vi "read.vi"(8 "error in (no error)":errorcluster, 10 "ILC":refnum<class "ILC.lvclass">, 11 "ReadILCTachometerStrategy in":refnum<class "ReadILCTachometerStrategy.lvclass">) -> (0 "error out":errorcluster, 2 "Value":dbl, 3 "ReadILCTachometerStrategy out":refnum<class "ReadILCTachometerStrategy.lvclass">)   [LabVIEW 2016, in "ReadILCTachometerStrategy.lvclass"]
uses:
  ReadILCTachometerStrategy.lvclass
  Common_ILC/ILC/ILC.lvclass
  Common_ILC/ILC/ILC.lvclass/ILC.ctl
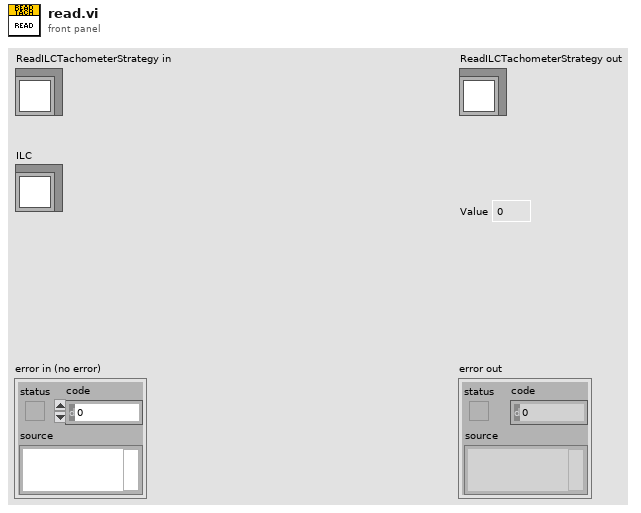
[diagram p1: front panel]
types:
  T1 = typedef "ILCCommon.lvlib/ILCTypedefs.lvlib/Inputs.ctl" = cluster{"Input Channels":T2, "Limit Switches":T3, "Tachometer":u16, "SSI Encoder":i32, "ADC":T4}
  T2 = typedef "ILCCommon.lvlib/ILCConfiguration.lvlib/Input Channels.ctl" = enum16{"Channel 0", "3 Channels", "5 Channels"}
  T3 = typedef "ILCCommon.lvlib/ILCTypedefs.lvlib/Limit Switches.ctl" = cluster{"1":bool, "2":bool}
  T4 = typedef "ILCCommon.lvlib/ILCTypedefs.lvlib/ADC Raw.ctl" = cluster{"Ch0":i32, "Ch1":i32, "Ch2":i32, "Ch3":i32, "Ch4":i32}
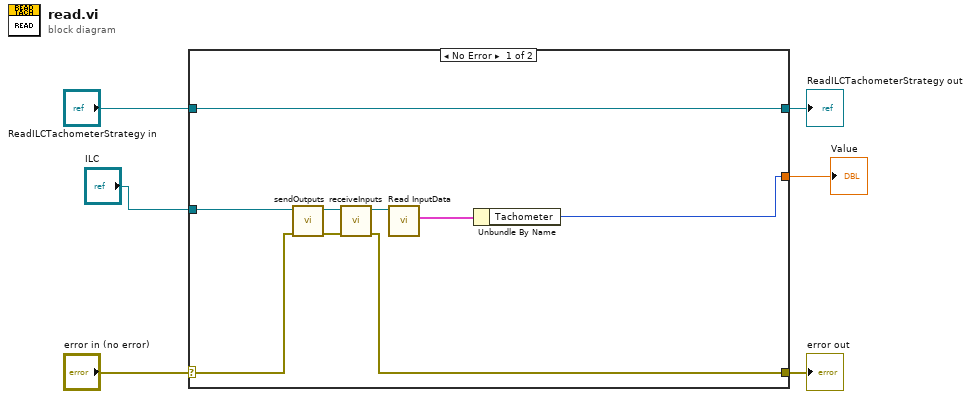
[diagram p0: block diagram]
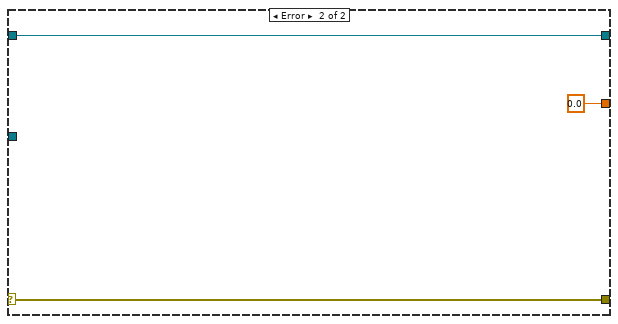
[diagram p2: hidden frame]
diagram:
  n1 = case shown="No Error" "error in (no error)" {
    selector: "error in (no error)" -> [w10 w18]
    tunnel: [w8 w18] -> w5
    tunnel: [w15 w17] -> w3
    tunnel: "ReadILCTachometerStrategy in" -> [w15 w17]
    tunnel: [w7 0.0 ("Value")] -> w2
    tunnel: "ILC" -> [w14 _]
    frame No Error {
      n2 = call "sendOutputs.vi"("error in (no error)"=w10, "ILC in"=w14) -> ("error out"=w9:errorcluster, "ILC out"=w13:refnum<class "ILC.lvclass">)  [unwired: 8 in]
      n3 = call "receiveInputs.vi"("error in (no error)"=w9, "ILC in"=w13) -> ("error out"=w8:errorcluster, "ILC out"=w12:refnum<class "ILC.lvclass">)  [unwired: 6 in, 2 out]
      n4 = call "Read InputData.vi"("ILC in"=w12) -> ("InputData"=w11:T1)  [unwired: 9 in, 1 out]
      n5 = Unbundle By Name(w11) -> ("Tachometer"=w7:u16)
    }
    frame Error {
    }
  }
  "error out" <- w5
  "ReadILCTachometerStrategy out" <- w3
  "Value" <- w2
